vi "replay_viewer.vi"() -> ()   [LabVIEW 2012]
uses:
  <vilib>/Utility/file.llb/Read From Spreadsheet File (string).vi
panel:
  out "Replay":string[][](array[string])
  out "End of chunk (s)":dbl
  out "Chunks over time":cluster{dbl[], dbl[]}(graph)
  out "Start of chunk (s)":dbl
  out "Chunk":string[][](array[string])
  in  "stop":bool
  in  "Select chunk":i32(slide) min=0 max=32 step=1 scale=0.0..32.0
  out "Times (s)":dbl[](array[numeric])
  in  "File path":path
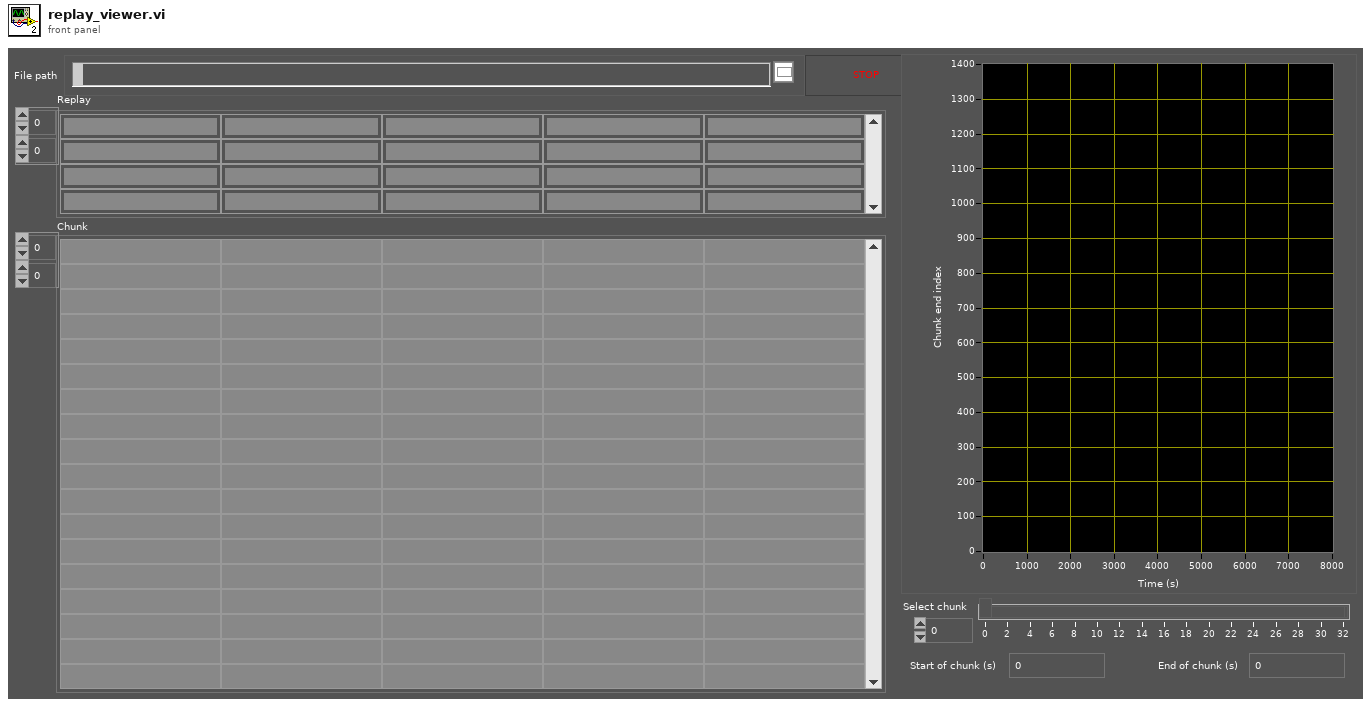
[diagram p1: front panel]
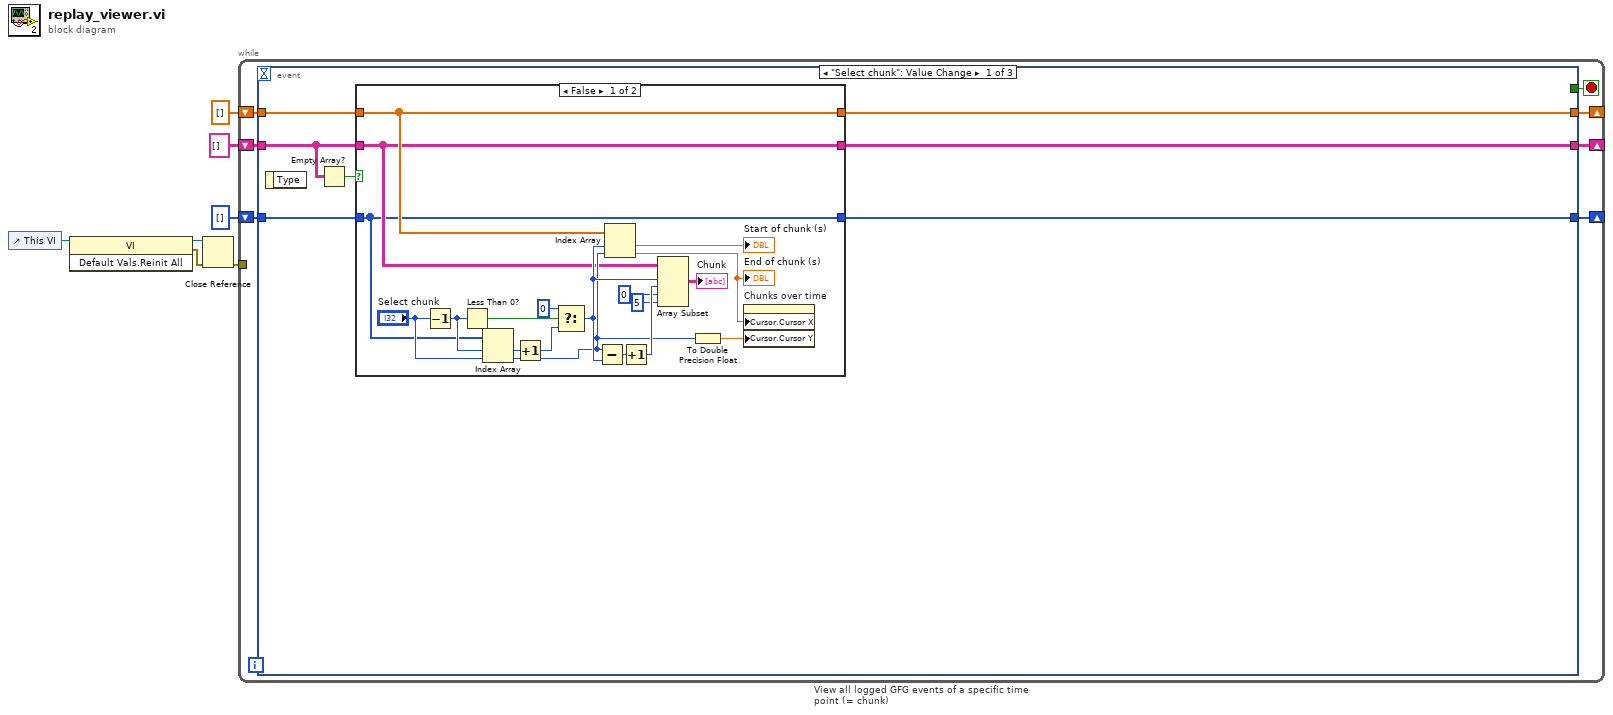
[diagram p0: block diagram]
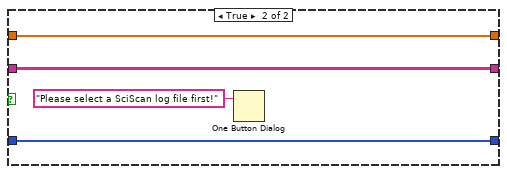
[diagram p2: hidden frame]
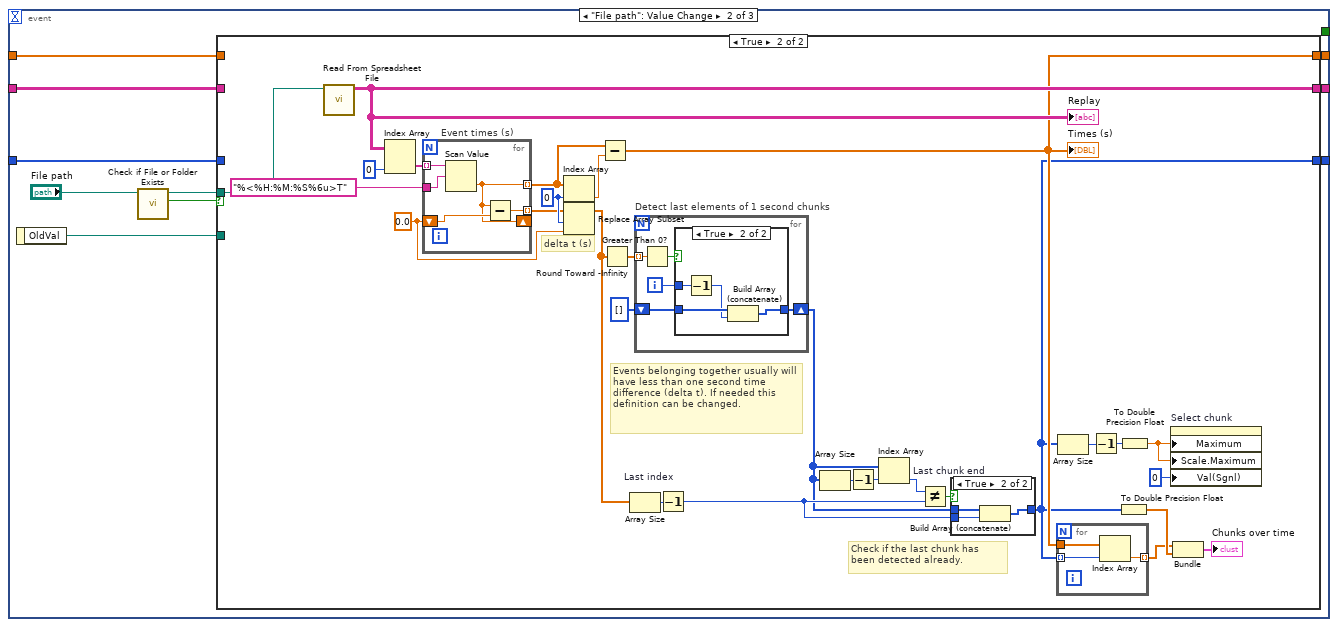
[diagram p3: hidden frame]
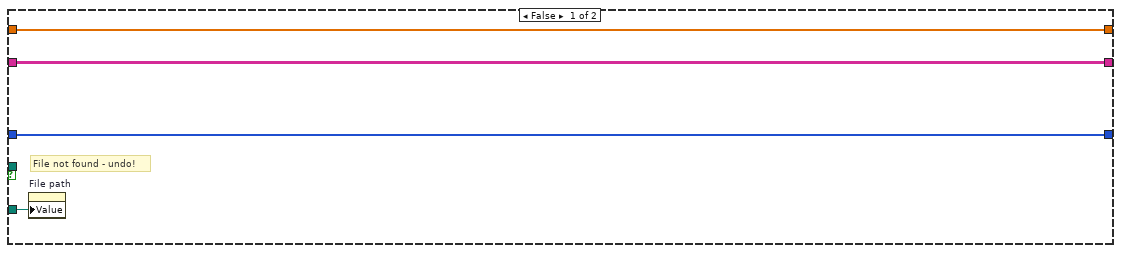
[diagram p4: hidden frame]
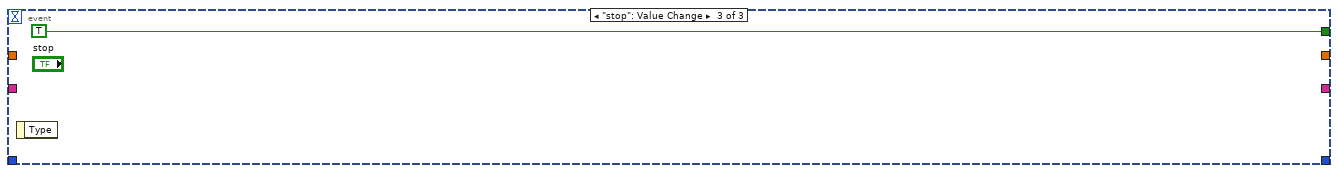
[diagram p7: hidden frame]
diagram:
  n1 = control-ref of="This VI"() -> (w2:refnum<vi>)
  n2 = invoke class="VI" method="Default Vals.Reinit All"(reference=w2) -> (reference out=w3:refnum<vi>, error out=w4:errorcluster)  [unwired: 2 in, 1 out]
  n3 = Close Reference(reference=w3, error in (no error)=w4) -> (error out=w1:errorcluster)
  n4 = while "View all logged GFG events of a specific time point (= chunk)" {
    shift-right: [w10] -> _
    shift-left: string[][] [] ("all rows") -> [w13]
    shift-right: [w9] -> _
    shift-left: dbl[] [] ("x-y") -> [w11]
    shift-right: [w8] -> _
    shift-left: i32[] [] -> [w12]
    tunnel: w1 -> [_]
    stop <- w14 stop-if-true
    n5 = event shown="[0] \"Select chunk\": Value Change" {
      selector: _ -> [_ _ _]
      dyn-events: _ -> [_ _ _]
      timeout: _ -> [_ _ _]
      tunnel: [_ _ TRUE ("stop")] -> w14
      tunnel: w13 -> [w19 w47 _]
      tunnel: w12 -> [w21 w45 _]
      tunnel: w11 -> [w20 w48 _]
      tunnel: [w16 w54 _] -> w10
      tunnel: [w17 w53 _] -> w9
      tunnel: [w15 w46 _] -> w8
      event "Select chunk": Value Change {
        n6 = event-data() -> ()  [unwired: 1 in, 1 out]
        n7 = Empty Array?(array=w19) -> (empty?=w18:bool)
        n8 = case shown="False" w18 {
          tunnel: w21 -> [w22 w41]
          tunnel: w20 -> [w24 w43]
          tunnel: w19 -> [w23 w42]
          tunnel: [w24 w43] -> w17
          tunnel: [w23 w42] -> w16
          tunnel: [w22 w41] -> w15
          frame False {
            n9 = Decrement(x="Select chunk") -> (x-1=w39:i32)
            n10 = Less Than 0?(x=w39) -> (x < 0?=w38:bool)
            n11 = Index Array(array=w22, index #1=w39, index #2="Select chunk") -> (element #1=w36:i32, element #2=w27:i32)
            n12 = Increment(x=w36) -> (x+1=w34:i32)
            n13 = Select(t=0 ("index"), s=w38, f=w34) -> (s? t:f=w28:i32)
            n14 = Subtract(x=w27, y=w28) -> (x-y=w33:i32)
            n15 = Index Array(array=w24, index #1=w28, index #2=w27) -> (element #1=→"Start of chunk (s)":dbl, element #2=w25:dbl)
            "End of chunk (s)" <- w25
            n16 = Increment(x=w33) -> (x+1=w32:i32)
            n17 = Array Subset(array=w23, index (row)=w28, length (row)=w32, index (col)=0 ("index"), length (col)=5 ("length")) -> (→"Chunk":string[][])
            n18 = To Double Precision Float(number=w27) -> (double precision float=w26:dbl)
            n19 = property on="Chunks over time" class="XYGraph (strict)"("Cursor.Cursor X"=w25, "Cursor.Cursor Y"=w26) -> ()  [unwired: 2 in, 2 out]
          }
          frame True {
            n20 = One Button Dialog(message="Please select a SciScan log file first!") -> ()  [unwired: 1 in, 1 out]
          }
        }
      }
      event "File path": Value Change {
        n21 = event-data() -> ("OldVal"=w49:path)  [unwired: 1 in]
        n22 = call <vilib>:"Check if File or Folder Exists.vi"("path"="File path") -> ("file or folder exists?"=w50:bool, "dup path"=w51:path)  [unwired: 8 in, 1 out]
        n23 = case shown="True" w50 {
          tunnel: [w56 w62] -> w54
          tunnel: [w57 w61] -> w53
          tunnel: w51 -> [_ w60]
          tunnel: w49 -> [w58 _]
          tunnel: w48 -> [w57 _]
          tunnel: w47 -> [w56 _]
          tunnel: [w55 w59] -> w46
          tunnel: w45 -> [w55 _]
          frame False {
            # "File not found - undo!"
            n24 = property on="File path" class="Path"("Value"=w58) -> ()  [unwired: 2 in, 2 out]
          }
          frame True {
            w69 = 0.0
            w70 = 0 ("index")
            # "Check if the last chunk has been detected already."
            # "Events belonging together usually will have less than one second time difference (delta t). If needed this definition can be changed."
            # "delta t (s)"
            n25 = call-poly <vilib>:"Read From Spreadsheet File.vi"("file path (dialog if empty)"=w60) -> ("all rows"=w62:string[][])  [unwired: 6 in, 4 out]
            "Replay" <- w62
            n26 = Index Array(array=w62, index (col)=0 ("disabled index (col)")) -> (element=w64:string[])  [unwired: 1 in]
            n27 = for "Event times (s)" {
              tunnel: w64 -> [w109] mode=indexing
              tunnel: [w105] -> w67 mode=indexing
              tunnel: "%<%H:%M:%S%6u>T" -> [w108]
              shift-right: [w105] -> _
              shift-left: w69 -> [w107]
              tunnel: [w106] -> w68 mode=indexing
              n28 = Scan Value(string=w109, format string=w108) -> (value=w105:dbl)  [unwired: 1 in, 1 out]
              n29 = Subtract(x=w105, y=w107) -> (x-y=w106:dbl)
            }
            n30 = Index Array(array=w67, index=w70) -> (element=w66:dbl)
            n31 = Replace Array Subset(array=w68, new element=w69, index=w70) -> (w76:dbl[])
            n32 = Subtract(x=w67, y=w66) -> (x-y=w61:dbl[])
            "Times (s)" <- w61
            n33 = Round Toward -Infinity(1:w76) -> (0:w71:dbl[])
            n34 = Array Size(array=w76) -> (size(s)=w77:i32)
            n35 = for "Detect last elements of 1 second chunks" {
              tunnel: w71 -> [w99] mode=indexing
              shift-right: [w95] -> w82
              shift-left: i32[] [] -> [w96]
              i -> [w97]
              n36 = Greater Than 0?(x=w99) -> (x > 0?=w98:bool)
              n37 = case shown="True" w98 {
                tunnel: w97 -> [_ w102]
                tunnel: w96 -> [w100 w104]
                tunnel: [w100 w103] -> w95
                frame False {
                }
                frame True {
                  n38 = Decrement(x=w102) -> (x-1=w101:i32)
                  n39 = Build Array (concatenate)(w104, w101) -> (w103:i32[])
                }
              }
            }
            n40 = Decrement "Last index"(x=w77) -> (x-1=w83:i32)
            n41 = Array Size(array=w82) -> (size(s)=w78:i32)
            n42 = Decrement(x=w78) -> (x-1=w79:i32)
            n43 = Index Array "Last chunk end"(array=w82, index=w79) -> (element=w80:i32)
            n44 = Not Equal?(x=w80, y=w83) -> (x != y?=w81:bool)
            n45 = case shown="True" w81 {
              tunnel: w82 -> [w91 w94]
              tunnel: w83 -> [_ w93]
              tunnel: [w91 w92] -> w59
              frame False {
              }
              frame True {
                n46 = Build Array (concatenate)(w94, w93) -> (w92:i32[])
              }
            }
            n47 = for {
              tunnel: w59 -> [w90] mode=indexing
              tunnel: w61 -> [w89]
              tunnel: [w88] -> w85 mode=indexing
              n48 = Index Array(array=w89, index=w90) -> (element=w88:dbl)
            }
            n49 = Array Size(array=w59) -> (size(s)=w73:i32)
            n50 = Decrement(x=w73) -> (x-1=w74:i32)
            n51 = To Double Precision Float(number=w59) -> (double precision float=w86:dbl[])
            n52 = To Double Precision Float(number=w74) -> (double precision float=w75:dbl)
            n53 = property on="Select chunk" class="Slide (strict)"("Maximum"=w75, "Scale.Maximum"=w75, "Val(Sgnl)"=0 ("Select chunk")) -> ()  [unwired: 2 in, 2 out]
            n54 = Bundle(w85, w86) -> (→"Chunks over time":cluster{dbl[], dbl[]})  [unwired: 1 in]
          }
        }
      }
      event "stop": Value Change {
        n55 = event-data() -> ()  [unwired: 1 in, 1 out]
      }
    }
  }
